vi "lickdetection.vi"() -> ()   [LabVIEW 2013]
uses:
  <vilib>/Analysis/NI_AALBase.lvlib
  <vilib>/ptbypt/NI_PtbyPt.lvlib
panel:
  out "standard deviation":dbl format="%0.2f"
  out "mean":dbl format="%0.2f"
  out "x .or. y?":bool
  in  "stop (F)":bool
  out "Waveform Chart":dynamicdata(graph)
  in  "stop":bool
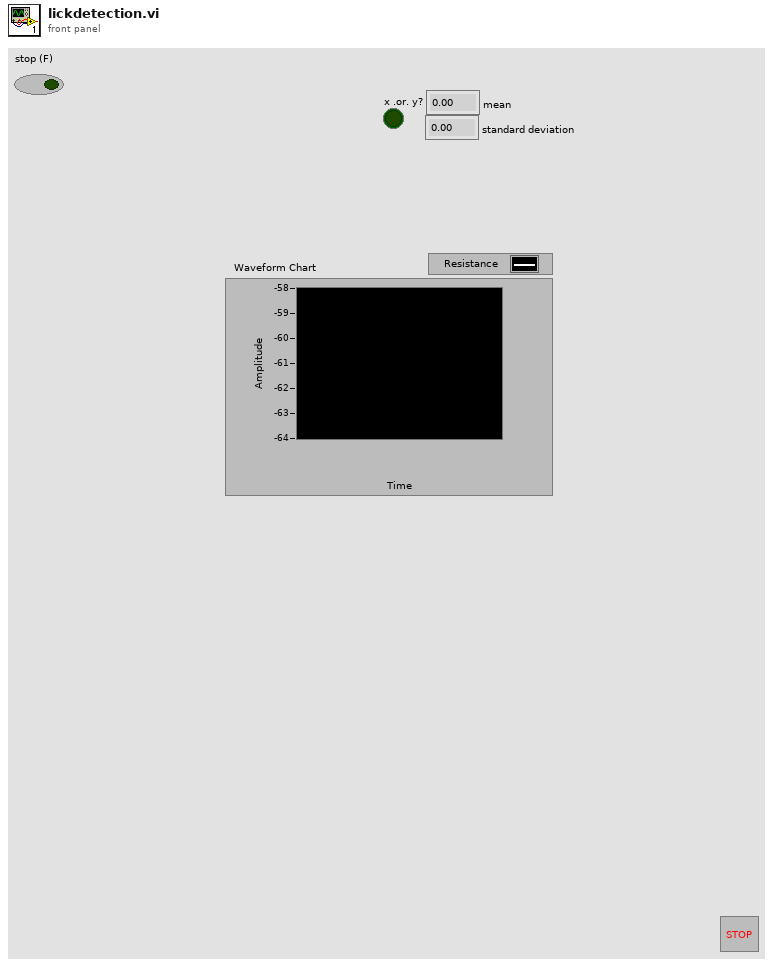
[diagram p1: front panel]
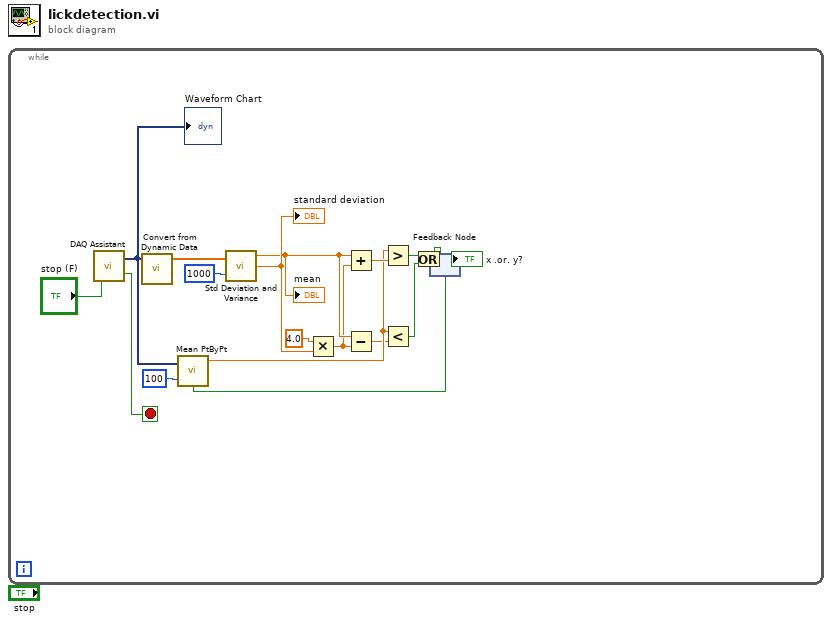
[diagram p0: block diagram]
diagram:
  n1 = while {
    stop <- w16 stop-if-true
    n2 = call "DAQ Assistant"("stop (F)"="stop (F)") -> ("data"=w14:dynamicdata, "stopped"=w16:bool)  [unwired: 15 in, 2 out]
    "Waveform Chart" <- w14
    n3 = call "Convert from Dynamic Data"("Dynamic Data Type"=w14) -> ("Array"=w13:dbl[])  [unwired: 3 in]
    n4 = call <vilib>:"Std Deviation and Variance.vi"("X"=w13, "Weighting (Sample)"=1000 ("sample length")) -> ("mean"=w7:dbl, "standard deviation"=w11:dbl)  [unwired: 1 out]
    "mean" <- w7
    "standard deviation" <- w11
    n5 = Multiply(x=4.0, y=w11) -> (x*y=w6:dbl)
    n6 = Add(x=w7, y=w6) -> (x+y=w9:dbl)
    n7 = Subtract(x=w7, y=w6) -> (x-y=w5:dbl)
    n8 = feedback #1() -> (w1:bool)  [unwired: 1 in]
    "x .or. y?" <- w1
    n9 = call <vilib>:"Mean PtByPt.vi"("x"=w14, "sample length"=100, "initialize"=w1) -> ("mean"=w8:dbl)  [unwired: 1 in, 1 out]
    n10 = Greater?(x=w8, y=w9) -> (0:w4:bool)
    n11 = Less?(x=w8, y=w5) -> (x < y?=w3:bool)
    n12 = Or(x=w4, y=w3) -> (x .or. y?=w2:bool)
    n13 = feedback-in #1(w2) -> ()
  }
